vi "KepcoDCPwr Configure Waveform Apply.vi"(0 "VISA Session":refnum<visa-resource-name>, 1 "List Type (DWell)":enum16{"Current List", "Voltage List"}(ring)=enum."Voltage List", 5 "Model In":string="BOP-HP", 7 "channel name (\"\")":string="\"\"", 9 "Waveform Type (Level)":T1(ring)=enum."Triangle", 11 "error in (no error)":errorcluster {"code" format="%.0x"}, 12 "Frequency":dbl, 13 "Amplidute":dbl, 14 "Offset":dbl) -> (4 "VISA Session Out":refnum<visa-resource-name>, 6 "Model Out":string, 8 "channel name out (\"\")":string="\"\"" caption="channel name Out (\"\")", 10 "Pointsl":i32 caption="Dwell", 15 "error out":errorcluster {"code" format="%.0x"})   [LabVIEW 2013]
doc: "This VI causes a waveform Segment to be added to an existing list.\n\nNote:\n\n1) This VI is available only for Advanced instruments (with an A at end of Model Number) or The BOP 1000 Watt.\n\nThere are 6 different types of segments supported by thei v.\n\nLEVEL and SLOPE requiring period @ frequency and level or end point at the offset.\n\nAll other types, Triangle, Sine, Ramp+ and Ramp- require the frequency, amplitude (PtoP) and offset ( the center point of the waveform segment."
uses:
  <vilib>/regexp/Match Regular Expression.xnode
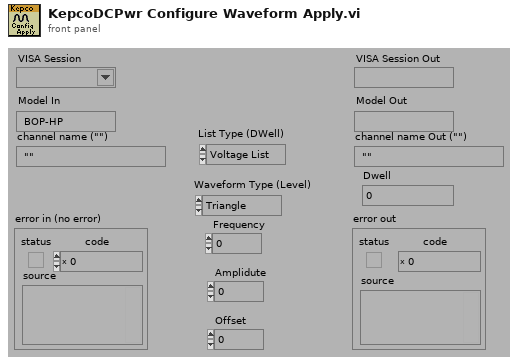
[diagram p1: front panel]
types:
  T1 = enum16{"Sine", "Triangle", "Sawtooth", "Dec Ramp", "Square", "Level", "Slope"}
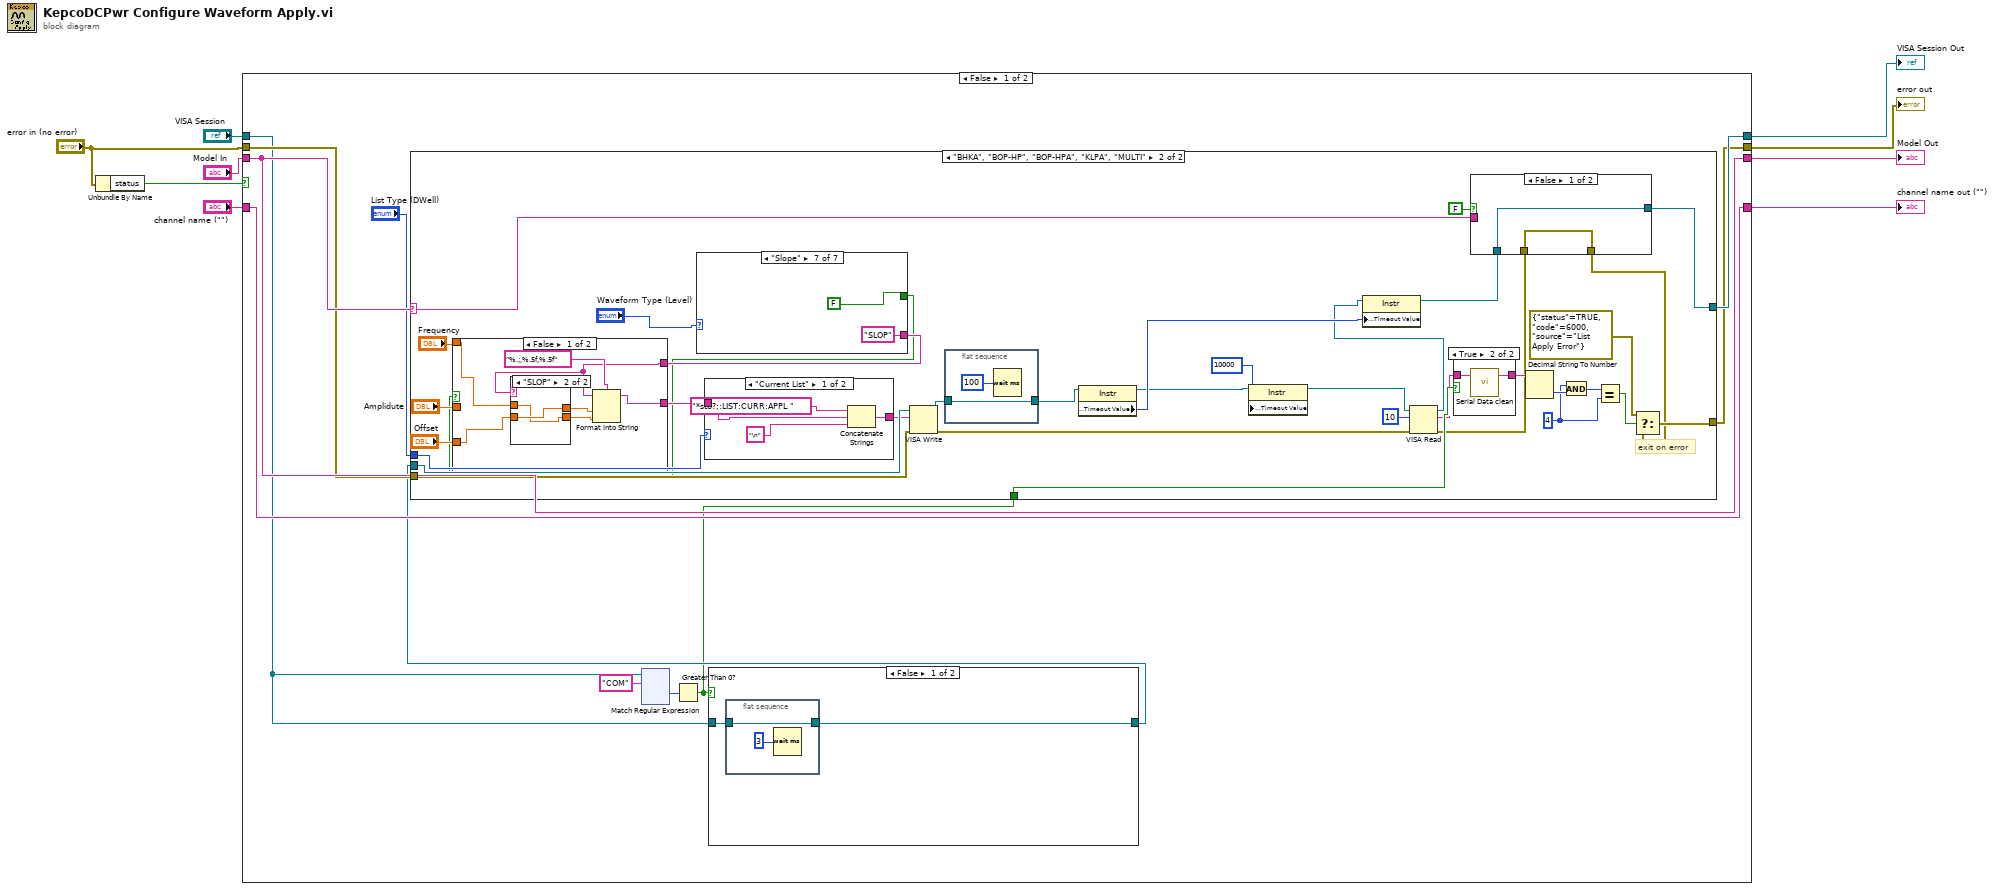
[diagram p0: block diagram]
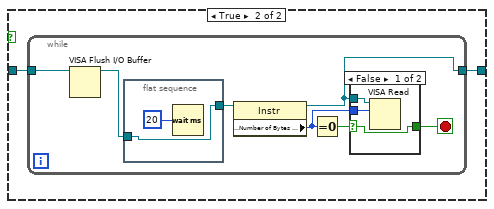
[diagram p2: hidden frame]
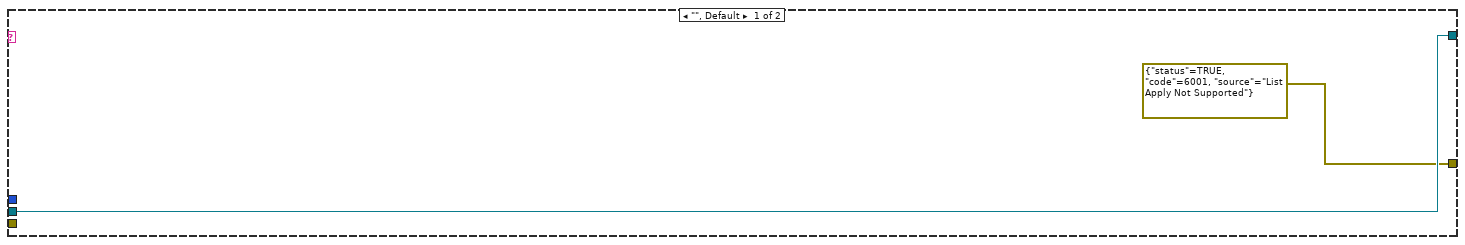
[diagram p4: hidden frame]
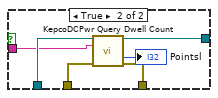
[diagram p5: hidden frame]
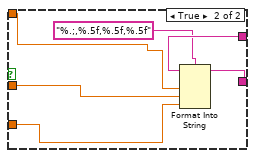
[diagram p7: hidden frame]
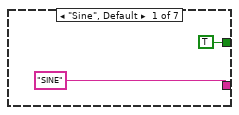
[diagram p8: hidden frame]
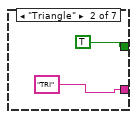
[diagram p9: hidden frame]
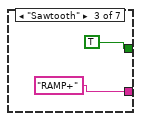
[diagram p10: hidden frame]
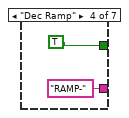
[diagram p11: hidden frame]
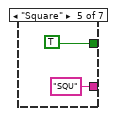
[diagram p12: hidden frame]
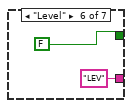
[diagram p13: hidden frame]
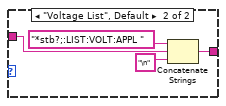
[diagram p15: hidden frame]
diagram:
  n1 = Unbundle By Name("error in (no error)") -> ("status"=w8:bool)
  n2 = case shown="False" w8 {
    tunnel: [w15 w242] -> w9
    tunnel: [w16 w243] -> w6
    tunnel: "VISA Session" -> [w11 w243]
    tunnel: "error in (no error)" -> [w18 w242]
    tunnel: [w19 w241] -> w3
    tunnel: "Model In" -> [w19 w241]
    tunnel: [w20 w240] -> w1
    tunnel: "channel name (\"\")" -> [w20 w240]
    frame False {
      n3 = xnode "Match Regular Expression"("input string"=w11, "regular expression"="COM") -> ("offset past match"=w13:i32)  [unwired: 2 in, 6 out]
      n4 = Greater Than 0?(x=w13) -> (x > 0?=w10:bool)
      n5 = case shown="False" w10 {
        tunnel: [w22 w26] -> w12
        tunnel: w11 -> [w21 w25]
        frame False {
          n6 = flat-sequence {
            tunnel: w21 -> [w24]
            tunnel: [w24] -> w22
            frame #0 {
              n7 = Wait (ms)(milliseconds to wait=u32 3 ("byte count (0)")) -> ()  [unwired: 1 out]
            }
          }
        }
        frame True {
          n8 = while {
            tunnel: w25 -> [w29]
            tunnel: [w31] -> w26
            stop <- w32 stop-if-true
            n9 = VISA Flush I/O Buffer(VISA resource name=w29) -> (VISA resource name out=w28:refnum<visa-resource-name>)  [unwired: 2 in, 1 out]
            n10 = flat-sequence {
              tunnel: w28 -> [w34]
              tunnel: [w34] -> w27
              frame #0 {
                n11 = Wait (ms)(milliseconds to wait=u32 20) -> ()  [unwired: 1 out]
              }
            }
            n12 = property class="Instr"(reference=w27) -> (reference out=w31:refnum<visa-resource-name>, "Serial Settings:Number of Bytes at Serial Port"=w30:u32)  [unwired: 1 in, 1 out]
            n13 = Equal To 0?(x=w30) -> (x = 0?=w33:bool)
            n14 = case shown="False" w33 {
              selector: w33 -> [w38 w39]
              tunnel: [w38 w39] -> w32
              tunnel: w31 -> [w37 _]
              tunnel: w30 -> [w36 _]
              frame False {
                n15 = VISA Read(VISA resource name=w37, byte count=w36) -> ()  [unwired: 1 in, 4 out]
              }
              frame True {
              }
            }
          }
        }
      }
      n16 = case shown="\"BHKA\", \"BOP-HP\", \"BOP-HPA\", \"KLPA\", \"MULTI\"" w19 {
        selector: w19 -> [_ w162]
        tunnel: w18 -> [_ w187]
        tunnel: w12 -> [w152 w186]
        tunnel: "List Type (DWell)" -> [_ w185]
        tunnel: [w152 w159] -> w16
        tunnel: [errorcluster {"status"=TRUE, "code"=6001, "source"="List Apply Not Supported"} ("t") w184] -> w15
        tunnel: w10 -> [_ w183]
        frame "", Default {
        }
        frame "BHKA", "BOP-HP", "BOP-HPA", "KLPA", "MULTI" {
          w175 = u16 4 ("y")
          # "exit on error"
          n17 = case shown="\"Slope\"" "Waveform Type (Level)" {
            tunnel: ["SINE" "TRI" "RAMP+" "RAMP-" "SQU" "LEV" "SLOP"] -> w164
            tunnel: [TRUE TRUE TRUE TRUE TRUE FALSE FALSE] -> w154
            frame "Sine", Default {
            }
            frame "Triangle" {
            }
            frame "Sawtooth" {
            }
            frame "Dec Ramp" {
            }
            frame "Square" {
            }
            frame "Level" {
            }
            frame "Slope" {
            }
          }
          n18 = case shown="False" w154 {
            tunnel: w164 -> [w200 w212]
            tunnel: [w201 w211] -> w158
            tunnel: "Frequency" -> [w197 w209]
            tunnel: "Amplidute" -> [_ w208]
            tunnel: "Offset" -> [w199 w207]
            frame False {
              n19 = case shown="\"SLOP\"" w200 {
                tunnel: [w203 w205] -> w198
                tunnel: w199 -> [w203 w206]
                tunnel: [w204 w206] -> w196
                tunnel: w197 -> [w204 w205]
                frame "False", Default {
                }
                frame "SLOP" {
                }
              }
              n20 = Format Into String(format string="%.;,%.5f,%.5f", initial string=w200, w196, w198) -> (resulting string=w201:string)  [unwired: 1 in, 1 out]
            }
            frame True {
              n21 = Format Into String(format string="%.;,%.5f,%.5f,%.5f", initial string=w212, w209, w208, w207) -> (resulting string=w211:string)  [unwired: 1 in, 1 out]
            }
          }
          n22 = case shown="\"Current List\"" w185 {
            tunnel: [w234 w239] -> w181
            tunnel: w158 -> [w232 w237]
            frame "Current List" {
              n23 = Concatenate Strings("*stb?;:LIST:CURR:APPL ", w232, "\n" ("string")) -> (w234:string)
            }
            frame "Voltage List", Default {
              n24 = Concatenate Strings("*stb?;:LIST:VOLT:APPL ", w237, "\n" ("string")) -> (w239:string)
            }
          }
          n25 = VISA Write(VISA resource name=w186, write buffer=w181, error in (no error)=w187) -> (VISA resource name out=w174:refnum<visa-resource-name>, error out=w179:errorcluster)  [unwired: 1 out]
          n26 = flat-sequence {
            tunnel: [w230] -> w167
            tunnel: w174 -> [w230]
            frame #0 {
              n27 = Wait (ms)(milliseconds to wait=u32 100) -> ()  [unwired: 1 out]
            }
          }
          n28 = property class="Instr"(reference=w167) -> (reference out=w169:refnum<visa-resource-name>, "General Settings:Timeout Value"=w170:u32)  [unwired: 1 in, 1 out]
          n29 = property class="Instr"(reference=w169, "General Settings:Timeout Value"=u32 10000) -> (reference out=w166:refnum<visa-resource-name>)  [unwired: 1 in, 1 out]
          n30 = VISA Read(VISA resource name=w166, byte count=u32 10, error in (no error)=w179) -> (VISA resource name out=w168:refnum<visa-resource-name>, read buffer=w173:string, error out=w161:errorcluster)  [unwired: 1 out]
          n31 = property class="Instr"(reference=w168, "General Settings:Timeout Value"=w170) -> (reference out=w163:refnum<visa-resource-name>)  [unwired: 1 in, 1 out]
          n32 = case shown="True" w183 {
            tunnel: w173 -> [w227 w228]
            tunnel: [w227 w229] -> w172
            frame False {
            }
            frame True {
              n33 = call "Serial Data clean.vi"("string"=w228) -> ("Stripped of Xon Xoff"=w229:string)  [unwired: 2 in]
            }
          }
          n34 = case shown="False" FALSE {
            tunnel: w163 -> [w189 w195]
            tunnel: w162 -> [_ w194]
            tunnel: w161 -> [w188 w193]
            tunnel: [w188 w192] -> w160
            tunnel: [w189 w191] -> w159
            frame False {
            }
            frame True {
              n35 = call "KepcoDCPwr Query Dwell Count.vi"("VISA Session"=w195, "Model In"=w194, "error in (no error)"=w193) -> ("VISA Session Out"=w191:refnum<visa-resource-name>, "voltage level"=→"Pointsl":i32, "error out"=w192:errorcluster)  [unwired: 8 in, 2 out]
            }
          }
          n36 = Decimal String To Number(string=w172) -> (number=w177:i32)  [unwired: 2 in, 1 out]
          n37 = And(x=w175, y=w177) -> (x .and. y?=w176:i32)
          n38 = Equal?(x=w176, y=w175) -> (x = y?=w182:bool)
          n39 = Select(t=errorcluster {"status"=TRUE, "code"=6000, "source"="List Apply Error"}, s=w182, f=w160) -> (s? t:f=w184:errorcluster)
        }
      }
    }
    frame True {
    }
  }
  "error out" <- w9
  "VISA Session Out" <- w6
  "channel name out (\"\")" <- w1
  "Model Out" <- w3
